vi "PV ActiveLine - Measurement Data Gauge 1 or 2.vi"(8 "Fehler (Eingang)":errorcluster, 10 "Sensor Nr.:":i32(ring) items=["sensor 1", "sensor 2"], 11 "Referenz in":refnum<visa-resource-name>) -> (0 "Cluster (Ausgang)":errorcluster, 1 "Pressure":dbl format="%.3e", 2 "Status":i32(ring) items=["data OK", "underrange", "overrange", "sensor error", "sensor off", "no sensor", "ID error"], 3 "Referenz out":refnum<visa-resource-name>)   [LabVIEW 2013, in "PV ActiveLine.lvlib"]
doc: "PRx - Measurement Data Gauge 1 or 2\n\nReceive: a,sx.xxxxEsxx\n\nStatus, a =\n0 –> Measurement data okay\n1 –> Underrange\n2 –> Overrange\n3 –> Sensor error\n4 –> Sensor off (IKR, PKR, IMR, PBR)\n5 –> No sensor (output: 5,2.0000E-2 [hPa])\n6 –> Identification error\n\nMeasurement value [in current pressure unit]\n\nValues always in exponential format. For logarithmic gauges, the 3rd and 4th decimal are always 0."
uses:
  <instrlib>/PV ActiveLine/PV ActiveLine.lvlib
panel:
  # "mbar"
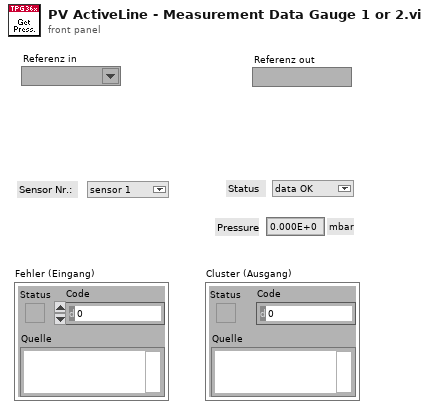
[diagram p1: front panel]
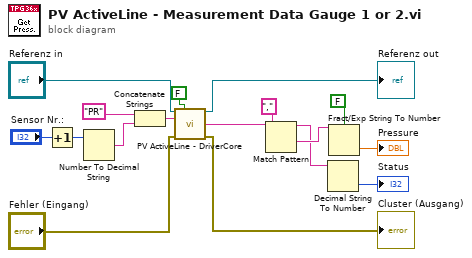
[diagram p0: block diagram]
diagram:
  n1 = Increment(x="Sensor Nr.:") -> (x+1=w16:i32)
  n2 = Number To Decimal String(number=w16) -> (decimal integer string=w12:string)  [unwired: 1 in]
  n3 = Concatenate Strings("PR", w12) -> (w7:string)
  n4 = call <instrlib>:"PV ActiveLine - DriverCore.vi"("Referenz in"="Referenz in", "Write/Read"=FALSE, "Command"=w7, "Fehler (Eingang)"="Fehler (Eingang)") -> ("Referenz out"=→"Referenz out":refnum<visa-resource-name>, "String Out"=w2:string, "Cluster (Ausgang)"=→"Cluster (Ausgang)":errorcluster)  [unwired: 9 in]
  n5 = Match Pattern(string=w2, regular expression=",") -> (before substring=w9:string, after substring=w10:string)  [unwired: 1 in, 2 out]
  n6 = Decimal String To Number(string=w9) -> (number=→"Status":i32)  [unwired: 2 in, 1 out]
  n7 = Fract/Exp String To Number(use system decimal point (T)=FALSE ("Systemdezimalzeichen verwenden (T)"), string=w10) -> (number=→"Pressure":dbl)  [unwired: 2 in, 1 out]
